vi "main.vi"() -> ()   [LabVIEW 2016]
uses:
  <vilib>/platform/TimedLoop/XDataNode/XDataNode.xnode
  <vilib>/Platform/TimedLoop/XDataNode/nitl_modes.ctl
  <vilib>/Platform/TimedLoop/XDataNode/XDNodeRunTimeDep.lvlib
  <vilib>/Platform/TimedLoop/XDataNode/wakeup.ctl
  <vilib>/Platform/TimedLoop/XDataNode/timing_clust.ctl
  <instrlib>/Lake Shore 425/Lake Shore 425.lvlib
panel:
  out "Temperature":dbl[](array[numeric])
  out "Multimeter":dbl[](array[numeric])
  out "Gaussmeter 3":dbl[](array[numeric])
  out "Gaussmeter 2":dbl[](array[numeric])
  out "Gaussmeter 1":dbl[](array[numeric])
  out "Status Multimeter":bool caption="Status"
  in  "Notes (must be entered before starting)":string
  in  "Multimeter\nMeasurement":u16(ring) caption="Measurement" items=["DC Voltage (50 A - 50 mV Shunt)", "DC Current (3 A Terminal)", "DC Current (10 A Terminal)", "AC Voltage (50 A - 50 mV Shunt)", "AC Current (3 A Terminal)", "AC Current (10 A Terminal)", "DC Voltage (other)", "AC Voltage (other)", "Continuity", "Diode", "Frequency", "Resistance 4-wire", "Period", "Resistance 2-wire", "Temperature", "DC Voltage Ratio", "Capacitance"]
  in  "VISA resource name Multimeter":refnum<visa-resource-name>
  in  "Switch Multimeter":bool
  out "Waveform Chart Multimeter":dbl(graph)
  in  "Temp. Monitor\nReadings per\nMeasurement":dbl caption="Temp. Monitor"
  in  "Multimeter\nReadings per\nMeasurement":dbl caption="Multimeter"
  in  "Readings per\nMeasurement":i32=5 caption="All Meters" min=1 step=1
  in  "Measure":bool
  out "z [mm]":dbl
  out "y [mm]":dbl
  out "x [mm]":dbl
  in  "Position File":path
  in  "Map Mode":bool
  in  "z":dbl caption="z [mm]"
  in  "y":dbl caption="y [mm]"
  in  "x":dbl caption="x [mm]"
  in  "Period [s]":dbl=1.0
  in  "Duration":dbl format="%<%H:%M:%S>t"
  out "XY Graph":cluster{dbl[], dbl[]}(graph)
  in  "Y-Axis":i32(ring)=6 items=["Time"=0, "x position"=1, "y position"=2, "z position"=3, "Gaussmeter 1"=4, "Gaussmeter 2"=6, "Gaussmeter 3"=8, "Multimeter"=10, "Temperature 1"=11, "Temperature 2"=12, "Temperature 3"=13, "Temperature 4"=14, "Temperature 5"=15, "Temperature 6"=16, "Temperature 7"=17, "Temperature 8"=18]
  in  "X-Axis":i32(ring)=4 items=["Time"=0, "x position"=1, "y position"=2, "z position"=3, "Gaussmeter 1"=4, "Gaussmeter 2"=6, "Gaussmeter 3"=8, "Multimeter"=10, "Temperature 1"=11, "Temperature 2"=12, "Temperature 3"=13, "Temperature 4"=14, "Temperature 5"=15, "Temperature 6"=16, "Temperature 7"=17, "Temperature 8"=18]
  in  "Moving Gaussmeter 3":bool caption="Moving"
  in  "x Gaussmeter 3":dbl caption="x [mm]"
  in  "y Gaussmeter 3":dbl caption="y [mm]"
  in  "z Gaussmeter 3":dbl caption="z [mm]"
  in  "Switch Gaussmeter 3":bool
  in  "VISA resource name Gaussmeter 3":refnum<visa-resource-name>
  out "Probe Type 3":u16(ring)=40 caption="Probe Type" items=["High Sensitivity"=40, "High Stability"=41, "Ultra-High Sensitivity"=42, "User Programmable Cable / High Sensitivity Probe"=50, "User Programmable Cable / High Stability Probe"=51, "User Programmable Cable / Ultra-High Sensitivity Probe"=52]
  out "Probe Serial Number 3":string caption="Probe Serial Number"
  out "Probe Sensitivity 3":dbl=0.001 caption="Probe Sensitivity" format="%^.3e"
  out "Field\nComp 3":bool caption="Field\nComp"
  out "Field Range  3":u16(ring)=1 caption="Field Range" items=["1 - Lowest"=1, "2"=2, "3"=3, "4 - Highest"=4]
  out "Field Units 3":u16(ring)=1 caption="Field Units" items=["Gauss"=1, "Tesla"=2, "Oersted"=3, "Amp/Meter"=4]
  out "Auto\nRange 3":bool caption="Auto\nRange"
  out "Status Gaussmeter 3":bool caption="Status"
  out "Waveform Chart Gaussmeter 3":dbl(graph)
  in  "Moving Gaussmeter 2":bool caption="Moving"
  in  "x Gaussmeter 2":dbl caption="x [mm]"
  in  "y Gaussmeter 2":dbl caption="y [mm]"
  in  "z Gaussmeter 2":dbl caption="z [mm]"
  in  "Switch Gaussmeter 2":bool
  in  "VISA resource name Gaussmeter 2":refnum<visa-resource-name>
  out "Probe Type 2":u16(ring)=40 caption="Probe Type" items=["High Sensitivity"=40, "High Stability"=41, "Ultra-High Sensitivity"=42, "User Programmable Cable / High Sensitivity Probe"=50, "User Programmable Cable / High Stability Probe"=51, "User Programmable Cable / Ultra-High Sensitivity Probe"=52]
  out "Probe Serial Number 2":string caption="Probe Serial Number"
  out "Probe Sensitivity 2":dbl=0.001 caption="Probe Sensitivity" format="%^.3e"
  out "Field\nComp 2":bool caption="Field\nComp"
  out "Field Range  2":u16(ring)=1 caption="Field Range" items=["1 - Lowest"=1, "2"=2, "3"=3, "4 - Highest"=4]
  out "Field Units 2":u16(ring)=1 caption="Field Units" items=["Gauss"=1, "Tesla"=2, "Oersted"=3, "Amp/Meter"=4]
  out "Auto\nRange 2":bool caption="Auto\nRange"
  out "Status Gaussmeter 2":bool caption="Status"
  out "Waveform Chart Gaussmeter 2":dbl(graph)
  in  "z Gaussmeter 1":dbl caption="z [mm]"
  in  "y Gaussmeter 1":dbl caption="y [mm]"
  in  "x Gaussmeter 1":dbl caption="x [mm]"
  in  "Moving Gaussmeter 1":bool caption="Moving"
  out "Status Gaussmeter 1":bool caption="Status"
  out "Auto\nRange":bool
  out "Field Units":u16(ring)=1 items=["Gauss"=1, "Tesla"=2, "Oersted"=3, "Amp/Meter"=4]
  out "Field Range":u16(ring)=1 items=["1 - Lowest"=1, "2"=2, "3"=3, "4 - Highest"=4]
  out "Field\nComp":bool
  out "Probe Sensitivity":dbl=0.001 format="%^.3e"
  out "Probe Serial Number":string
  out "Probe Type":u16(ring)=40 items=["High Sensitivity"=40, "High Stability"=41, "Ultra-High Sensitivity"=42, "User Programmable Cable / High Sensitivity Probe"=50, "User Programmable Cable / High Stability Probe"=51, "User Programmable Cable / Ultra-High Sensitivity Probe"=52]
  in  "VISA resource name Gaussmeter 1":refnum<visa-resource-name>
  in  "Switch Gaussmeter 1":bool
  out "Waveform Chart Gaussmeter 1":dbl(graph)
  out "Time [s]":dbl
  in  "Stop Button":bool
  out "Output File Name":string
  out "Output File Path":path
  in  "Output Folder Path":path=path "C:/Users/ephenix/Dropbox/Stony Brook Research Team Folder/LabVIEW/DATA_MegaVIEW"
  in  "VISA resource name Temperature Monitor":refnum<visa-resource-name>
  in  "Switch Temperature Monitor":bool
  out "Waveform Chart Temperature Monitor":dbl(graph)
  # "Multimeter (Agilent 34461A)"
  # "Readings per"
  # "Measurement"
  # "Timed MeasurementSettings"
  # "XY Graph Axes"
  # "Gaussmeter 3 (Lake Shore 425)"
  # "Gaussmeter 2 (Lake Shore 425)"
  # "Gaussmeter 1 (Lake Shore 425)"
  # "Temperature Monitor (Lake Shore 218)"
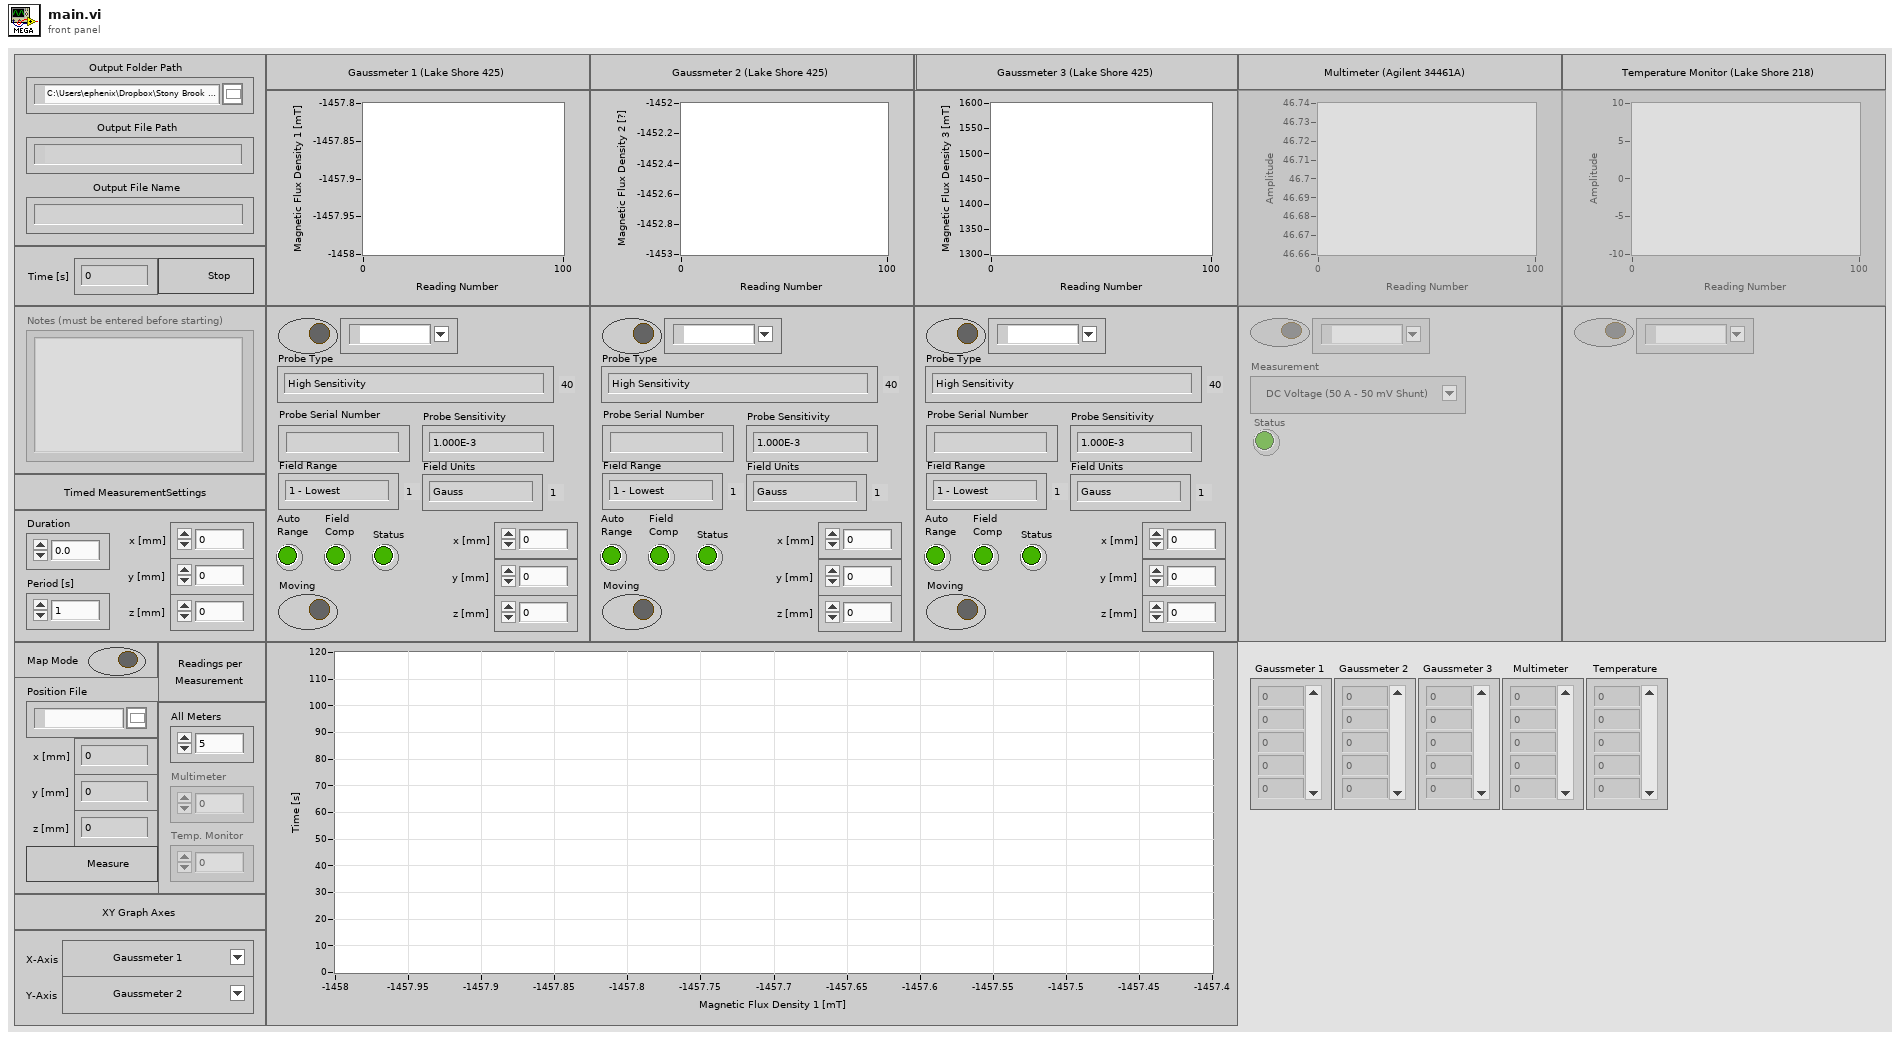
[diagram p1: front panel]
types:
  T1 = enum8{"Enabled", "Disabled", "Disabled and Grayed Out"}
  T2 = cluster{"VISA recourse name":refnum<visa-resource-name>, "switch":bool, "text":string, "units":i32, "status":bool}
  T3 = cluster{"VISA recourse name":cluster{refnum<visa-resource-name>, refnum<visa-resource-name>, refnum<visa-resource-name>, refnum<visa-resource-name>, refnum<visa-resource-name>}, "switch":cluster{bool, bool, bool, bool, bool}, "text":cluster{string, string, string, string, string}, "units":cluster{i32, i32, i32, i32, i32}}
  T4 = cluster{"VISA recourse name":refnum<visa-resource-name>, "VISA recourse name":refnum<visa-resource-name>, "VISA recourse name":refnum<visa-resource-name>, "VISA recourse name":refnum<visa-resource-name>, "VISA recourse name":refnum<visa-resource-name>}
  T5 = cluster{"switch":bool, "switch":bool, "switch":bool, "switch":bool, "switch":bool}
  T6 = cluster{"text":string, "text":string, "text":string, "text":string, "text":string}
  T7 = cluster{"units":i32, "units":i32, "units":i32, "units":i32, "units":i32}
  T8 = enum16{"open", "replace", "create", "open or create", "replace or create", "replace or create with confirmation"}
  T9 = typedef "XDNodeRunTimeDep.lvlib/timing_clust.ctl" = cluster{"Expected End [f-1]":u64, "Actual End [f-1]":u64, "Finished Late? [f-1]":bool, "Expected End [i-1]":u64, "Actual End [i-1]":u64, "Finished Late? [i-1]":bool, "Expected Start [i]":u64, "Actual Start [i]":u64, "Expected Start [f]":u64, "Actual Start [f]":u64, "Source Name":string, "Structure Name":string, "Period":i64, "Deadline":i64, "Offset":i64, "Start":i64, "Priority":i32, "Timeout":i32, "Mode":T10, "Wakeup Reason":T11, "Error":errorcluster, "Source Type":string, "Secondary Source Type":string, "Global End Time":u64, "Global Start Time":u64, "Frame Duration":u64, "Iteration Duration":u64, "Assigned CPU":i32, "I/O Scan Engine Mode":u32}
  T10 = typedef "XDNodeRunTimeDep.lvlib/nitl_modes.ctl" = enum32{"No Change", "Process missed periods, maintain original phase", "Discard missed periods, maintain original phase", "Process missed periods, ignore original phase", "Discard missed periods, ignore original phase"}
  T11 = typedef "XDNodeRunTimeDep.lvlib/wakeup.ctl" = enum32{"Normal", "Aborted", "Asynchronous wakeup", "Timing source error", "Timed loop error", "Timeout"}
  T12 = cluster{refnum<visa-resource-name>, refnum<visa-resource-name>, refnum<visa-resource-name>, refnum<visa-resource-name>, refnum<visa-resource-name>}
  T13 = cluster{"Field Reading":dbl, "Field Reading":dbl, "Field Reading":dbl, "Reading":dbl}
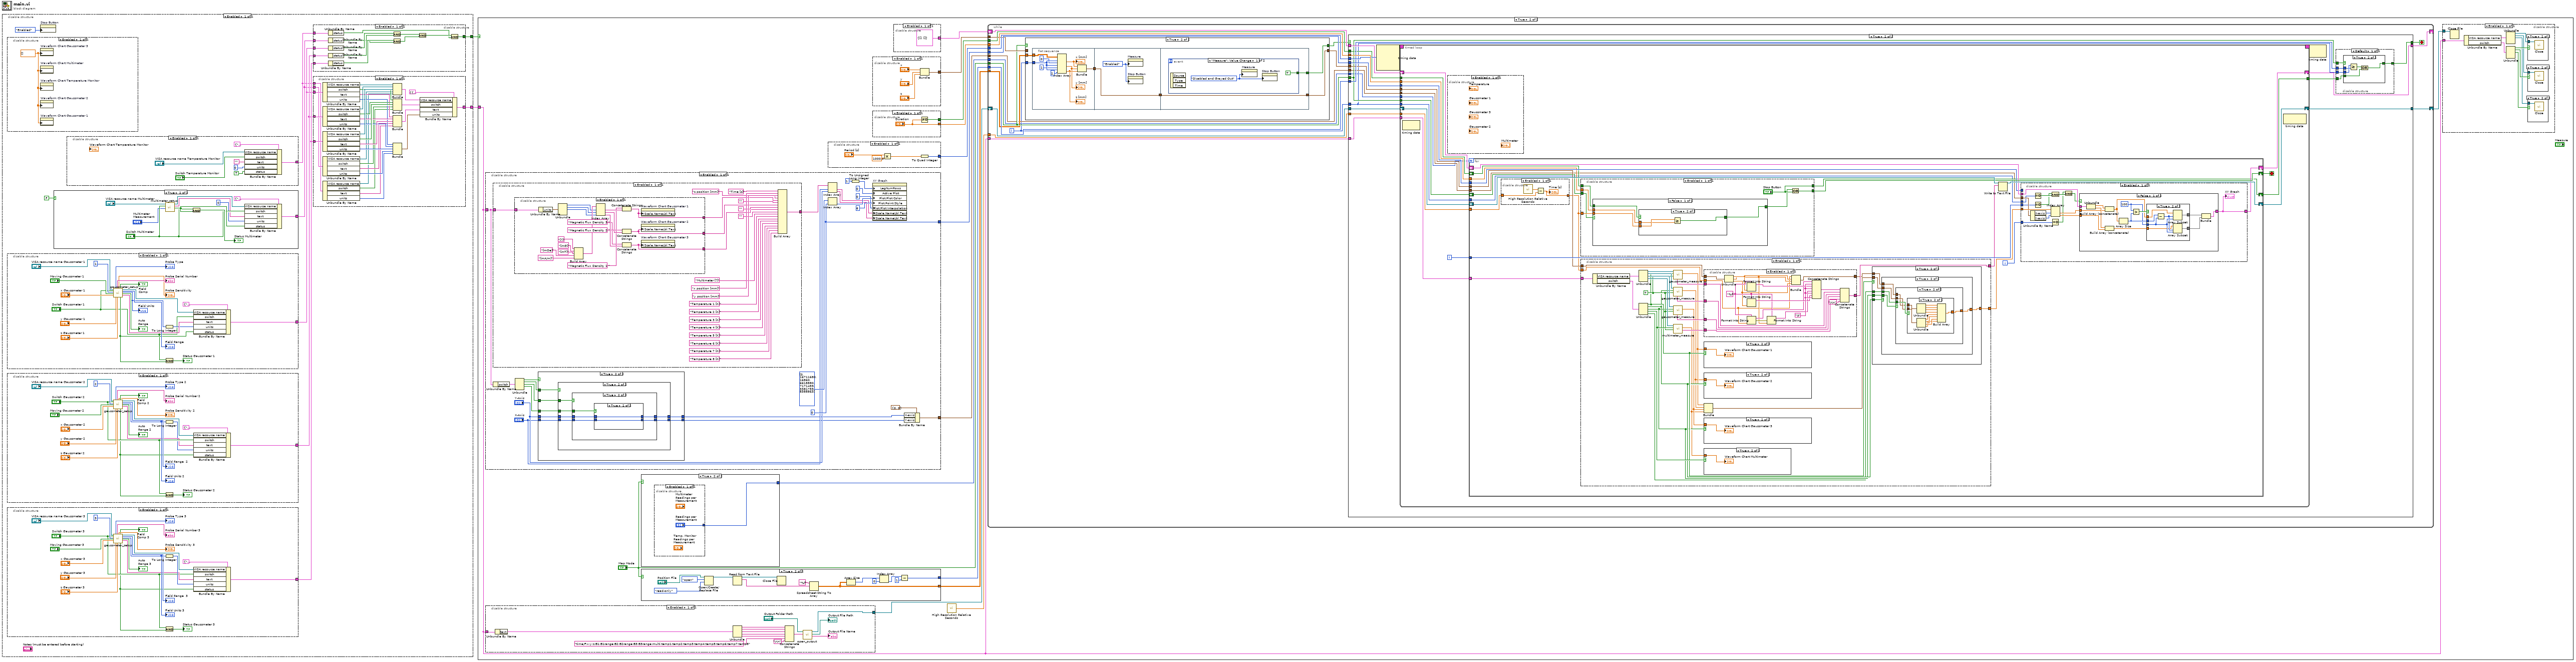
[diagram p0: block diagram]
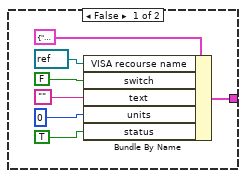
[diagram p2: hidden frame]
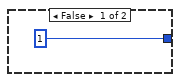
[diagram p4: hidden frame]
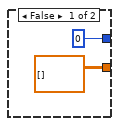
[diagram p12: hidden frame]
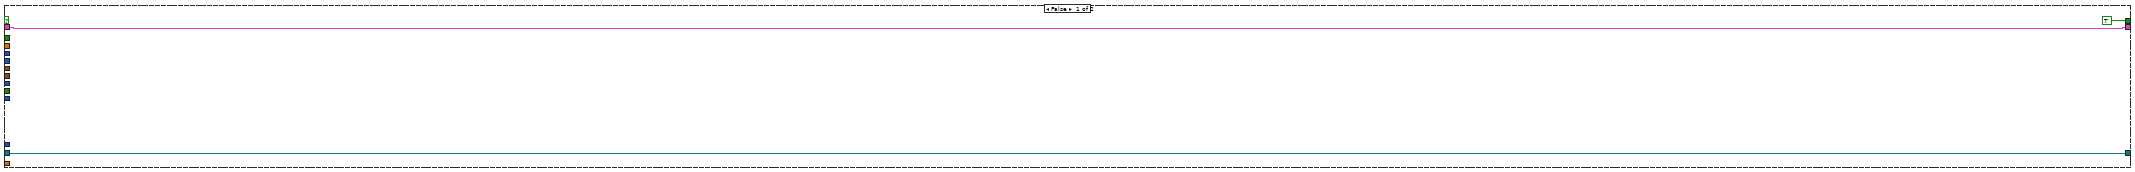
[diagram p13: hidden frame]
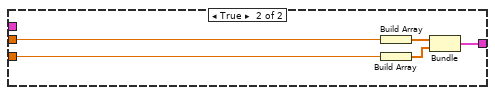
[diagram p15: hidden frame]
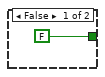
[diagram p16: hidden frame]
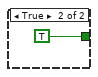
[diagram p17: hidden frame]
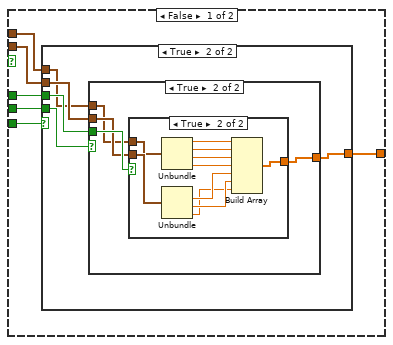
[diagram p18: hidden frame]
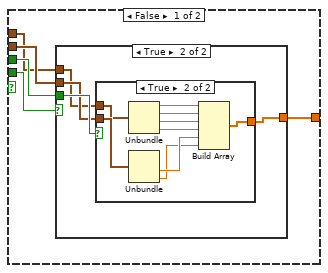
[diagram p19: hidden frame]
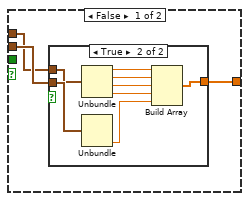
[diagram p20: hidden frame]
diagram:
  n1 = disable-structure shown="Enabled" {
    disable-tunnel: [w11] -> w2
    disable-tunnel: [w10] -> w1
    frame Enabled {
      n2 = disable-structure shown="Enabled" {
        frame Enabled {
          w36 = dbl[] [] ("History Data")
          n3 = property on="Waveform Chart Gaussmeter 3" class="WFChart (strict)"("History Data"=w36) -> ()  [unwired: 2 in, 2 out]
          n4 = property on="Waveform Chart Multimeter" class="WFChart (strict)"("History Data"=w36) -> ()  [unwired: 2 in, 2 out]
          n5 = property on="Waveform Chart Temperature Monitor" class="WFChart (strict)"("History Data"=w36) -> ()  [unwired: 2 in, 2 out]
          n6 = property on="Waveform Chart Gaussmeter 2" class="WFChart (strict)"("History Data"=w36) -> ()  [unwired: 2 in, 2 out]
          n7 = property on="Waveform Chart Gaussmeter 1" class="WFChart (strict)"("History Data"=w36) -> ()  [unwired: 2 in, 2 out]
        }
      }
      n8 = disable-structure shown="Enabled" {
        disable-tunnel: [w82] -> w8
        frame Enabled {
          n9 = call "gaussmeter_setup.vi"("VISA resource name Gaussmeter"="VISA resource name Gaussmeter 1", "Switch Gaussmeter"="Switch Gaussmeter 1", "Gaussmeter Number"=u8 1, "Moving Gaussmeter"="Moving Gaussmeter 1", "x Gaussmeter"="x Gaussmeter 1", "y Gaussmeter"="y Gaussmeter 1", "z Gaussmeter"="z Gaussmeter 1") -> ("Probe Type"=→"Probe Type":u16, "Probe Serial Number"=→"Probe Serial Number":string, "Probe Sensitivity"=→"Probe Sensitivity":dbl, "Probe Field\nCompensation On"=→"Field\nComp":bool, "Status Gaussmeter"=w80:bool, "Gaussmeter VISA resource name out"=w85:refnum<visa-resource-name>, "Field Range"=→"Field Range":u16, "Field Units"=w86:u16, "Auto Range On"=→"Auto\nRange":bool, "Text Output"=w84:string)  [unwired: 2 in, 1 out]
          "Field Units" <- w86
          n10 = To Long Integer(number=w86) -> (32bit integer=w83:i32)
          n11 = And(x="Switch Gaussmeter 1", y=w80) -> (x .and. y?=→"Status Gaussmeter 1":bool)
          n12 = Bundle By Name(cluster=T2 {"VISA recourse name"="", "switch"=TRUE, "text"="", "units"=0, "status"=TRUE} ("input cluster"), "VISA recourse name"=w85, "switch"="Switch Gaussmeter 1", "text"=w84, "units"=w83, "status"=w80) -> (w82:T2)
        }
      }
      n13 = disable-structure shown="Enabled" {
        disable-tunnel: [w58] -> w7
        frame Enabled {
          n14 = call "gaussmeter_setup.vi"("VISA resource name Gaussmeter"="VISA resource name Gaussmeter 2", "Switch Gaussmeter"="Switch Gaussmeter 2", "Gaussmeter Number"=u8 2, "Moving Gaussmeter"="Moving Gaussmeter 2", "x Gaussmeter"="x Gaussmeter 2", "y Gaussmeter"="y Gaussmeter 2", "z Gaussmeter"="z Gaussmeter 2") -> ("Probe Type"=→"Probe Type 2":u16, "Probe Serial Number"=→"Probe Serial Number 2":string, "Probe Sensitivity"=→"Probe Sensitivity 2":dbl, "Probe Field\nCompensation On"=→"Field\nComp 2":bool, "Status Gaussmeter"=w59:bool, "Gaussmeter VISA resource name out"=w63:refnum<visa-resource-name>, "Field Range"=→"Field Range  2":u16, "Field Units"=w65:u16, "Auto Range On"=→"Auto\nRange 2":bool, "Text Output"=w61:string)  [unwired: 2 in, 1 out]
          "Field Units 2" <- w65
          n15 = To Long Integer(number=w65) -> (32bit integer=w60:i32)
          n16 = And(x="Switch Gaussmeter 2", y=w59) -> (x .and. y?=→"Status Gaussmeter 2":bool)
          n17 = Bundle By Name(cluster=T2 {"VISA recourse name"="", "switch"=TRUE, "text"="", "units"=0, "status"=TRUE} ("input cluster"), "VISA recourse name"=w63, "switch"="Switch Gaussmeter 2", "text"=w61, "units"=w60, "status"=w59) -> (w58:T2)
        }
      }
      n18 = disable-structure shown="Enabled" {
        disable-tunnel: [w37] -> w9
        frame Enabled {
          n19 = call "gaussmeter_setup.vi"("VISA resource name Gaussmeter"="VISA resource name Gaussmeter 3", "Switch Gaussmeter"="Switch Gaussmeter 3", "Gaussmeter Number"=u8 3, "Moving Gaussmeter"="Moving Gaussmeter 3", "x Gaussmeter"="x Gaussmeter 3", "y Gaussmeter"="y Gaussmeter 3", "z Gaussmeter"="z Gaussmeter 3") -> ("Probe Type"=→"Probe Type 3":u16, "Probe Serial Number"=→"Probe Serial Number 3":string, "Probe Sensitivity"=→"Probe Sensitivity 3":dbl, "Probe Field\nCompensation On"=→"Field\nComp 3":bool, "Status Gaussmeter"=w38:bool, "Gaussmeter VISA resource name out"=w41:refnum<visa-resource-name>, "Field Range"=→"Field Range  3":u16, "Field Units"=w44:u16, "Auto Range On"=→"Auto\nRange 3":bool, "Text Output"=w42:string)  [unwired: 2 in, 1 out]
          "Field Units 3" <- w44
          n20 = To Long Integer(number=w44) -> (32bit integer=w43:i32)
          n21 = And(x="Switch Gaussmeter 3", y=w38) -> (x .and. y?=→"Status Gaussmeter 3":bool)
          n22 = Bundle By Name(cluster=T2 {"VISA recourse name"="", "switch"=TRUE, "text"="", "units"=0, "status"=TRUE} ("input cluster"), "VISA recourse name"=w41, "switch"="Switch Gaussmeter 3", "text"=w42, "units"=w43, "status"=w38) -> (w37:T2)
        }
      }
      n23 = property on="Stop Button" class="Bool"("DisabledEnum"=T1."Enabled" ("Disabled")) -> ()  [unwired: 2 in, 2 out]
      n24 = case shown="True" FALSE {
        tunnel: [w17 w19] -> w5
        frame False {
          n25 = Bundle By Name(cluster=T2 {"VISA recourse name"="", "switch"=TRUE, "text"="", "units"=0, "status"=TRUE} ("input cluster"), "VISA recourse name"=refnum<visa-resource-name> refnum, "switch"=FALSE, "text"="", "units"=0, "status"=TRUE) -> (w17:T2)
        }
        frame True {
          n26 = call "multimeter_setup.vi"("Measurement"="Multimeter\nMeasurement", "Switch"="Switch Multimeter", "VISA resource name"="VISA resource name Multimeter") -> ("status"=w27:bool, "text"=w23:string, "VISA resource name out"=w22:refnum<visa-resource-name>)  [unwired: 5 in, 1 out]
          n27 = And(x="Switch Multimeter", y=w27) -> (x .and. y?=→"Status Multimeter":bool)
          n28 = Bundle By Name(cluster=T2 {"VISA recourse name"="", "switch"=TRUE, "text"="", "units"=0, "status"=TRUE} ("input cluster"), "VISA recourse name"=w22, "switch"="Switch Multimeter", "text"=w23, "units"=0, "status"=w27) -> (w19:T2)
        }
      }
      n29 = disable-structure shown="Enabled" {
        disable-tunnel: [w32] -> w6
        frame Enabled {
          n30 = Bundle By Name(cluster=T2 {"VISA recourse name"="", "switch"=TRUE, "text"="", "units"=0, "status"=TRUE} ("input cluster"), "VISA recourse name"="VISA resource name Temperature Monitor", "switch"="Switch Temperature Monitor", "text"="", "units"=0, "status"=TRUE) -> (w32:T2)
        }
      }
      n31 = disable-structure shown="Enabled" {
        disable-tunnel: [w131] -> w11
        disable-tunnel: w9 -> [w139]
        disable-tunnel: w8 -> [w143]
        disable-tunnel: w7 -> [w140]
        disable-tunnel: w6 -> [w137]
        disable-tunnel: w5 -> [w138]
        frame Enabled {
          n32 = Unbundle By Name(w137) -> ("status"=w132:bool)
          n33 = Unbundle By Name(w138) -> ("status"=w135:bool)
          n34 = Unbundle By Name(w143) -> ("status"=w141:bool)
          n35 = Unbundle By Name(w140) -> ("status"=w142:bool)
          n36 = Unbundle By Name(w139) -> ("status"=w136:bool)
          n37 = And(x=w141, y=w142) -> (x .and. y?=w144:bool)
          n38 = And(x=w136, y=w135) -> (x .and. y?=w134:bool)
          n39 = And(x=w144, y=w134) -> (x .and. y?=w133:bool)
          n40 = And(x=w133, y=w132) -> (x .and. y?=w131:bool)
        }
      }
      n41 = disable-structure shown="Enabled" {
        disable-tunnel: [w126] -> w10
        disable-tunnel: w8 -> [w125]
        disable-tunnel: w7 -> [w123]
        disable-tunnel: w9 -> [w124]
        disable-tunnel: w5 -> [w109]
        disable-tunnel: w6 -> [w108]
        frame Enabled {
          n42 = Unbundle By Name(w125) -> ("VISA recourse name"=w122:refnum<visa-resource-name>, "switch"=w118:bool, "text"=w116:string, "units"=w111:i32)
          n43 = Unbundle By Name(w123) -> ("VISA recourse name"=w121:refnum<visa-resource-name>, "switch"=w119:bool, "text"=w115:string, "units"=w112:i32)
          n44 = Unbundle By Name(w124) -> ("VISA recourse name"=w120:refnum<visa-resource-name>, "switch"=w117:bool, "text"=w114:string, "units"=w113:i32)
          n45 = Unbundle By Name(w109) -> ("VISA recourse name"=w100:refnum<visa-resource-name>, "switch"=w103:bool, "text"=w104:string, "units"=w107:i32)
          n46 = Unbundle By Name(w108) -> ("VISA recourse name"=w101:refnum<visa-resource-name>, "switch"=w102:bool, "text"=w105:string, "units"=w106:i32)
          n47 = Bundle("VISA recourse name"=w122, "VISA recourse name"=w121, "VISA recourse name"=w120, "VISA recourse name"=w100, "VISA recourse name"=w101) -> (w130:T4)  [unwired: 1 in]
          n48 = Bundle("switch"=w118, "switch"=w119, "switch"=w117, "switch"=w103, "switch"=w102) -> (w129:T5)  [unwired: 1 in]
          n49 = Bundle("text"=w116, "text"=w115, "text"=w114, "text"=w104, "text"=w105) -> (w128:T6)  [unwired: 1 in]
          n50 = Bundle("units"=w111, "units"=w112, "units"=w113, "units"=w107, "units"=w106) -> (w127:T7)  [unwired: 1 in]
          n51 = Bundle By Name(cluster=T3 {"VISA recourse name"={"", "", "", "", ""}, "switch"={TRUE, TRUE, TRUE, TRUE, TRUE}, "text"={"", "", "", "", ""}, "units"={0, 0, 0, 0, 0}}, "VISA recourse name"=w130, "switch"=w129, "text"=w128, "units"=w127) -> (w126:T3)
        }
      }
    }
  }
  n52 = case shown="True" w2 {
    tunnel: w1 -> [_ w150]
    frame False {
    }
    frame True {
      n53 = disable-structure shown="Enabled" {
        disable-tunnel: [w208] -> w155
        disable-tunnel: w150 -> [w195]
        disable-tunnel: [w196] -> w151
        frame Enabled {
          w208 = 0
          n54 = disable-structure shown="Enabled" {
            disable-tunnel: [w245] -> w198
            disable-tunnel: w195 -> [w229]
            frame Enabled {
              n55 = disable-structure shown="Enabled" {
                disable-tunnel: [w257] -> w232
                disable-tunnel: [w256] -> w231
                disable-tunnel: [w255] -> w230
                disable-tunnel: w229 -> [w254]
                frame Enabled {
                  n56 = Unbundle By Name(w254) -> ("units"=w253:cluster{i32, i32, i32, i32, i32})
                  n57 = Unbundle(w253) -> (w252:i32, w251:i32, w250:i32)  [unwired: 2 out]
                  n58 = Build Array("[?]", "[mG]", "[mT]", "[mOe]", "[mA/m]") -> (w264:string[])
                  n59 = Index Array(array=w264, index #1=w252, index #2=w251, index #3=w250) -> (element #1=w261:string, element #2=w262:string, element #3=w263:string)
                  n60 = Concatenate Strings("Magnetic Flux Density 1 ", w261) -> (w255:string)
                  n61 = Concatenate Strings("Magnetic Flux Density 2 ", w262) -> (w256:string)
                  n62 = Concatenate Strings("Magnetic Flux Density 3 ", w263) -> (w257:string)
                  n63 = property on="Waveform Chart Gaussmeter 1" class="WFChart (strict)"("YScale.NameLbl.Text"=w255) -> ()  [unwired: 2 in, 2 out]
                  n64 = property on="Waveform Chart Gaussmeter 2" class="WFChart (strict)"("YScale.NameLbl.Text"=w256) -> ()  [unwired: 2 in, 2 out]
                  n65 = property on="Waveform Chart Gaussmeter 3" class="WFChart (strict)"("YScale.NameLbl.Text"=w257) -> ()  [unwired: 2 in, 2 out]
                }
              }
              n66 = Build Array("Time [s]", "x position [mm]", "y position [mm]", "z position [mm]", w230, "", w231, "", w232, "", "Multimeter [?]", "Temperature 1 [K]", "Temperature 2 [K]", "Temperature 3 [K]", "Temperature 4 [K]", "Temperature 5 [K]", "Temperature 6 [K]", "Temperature 7 [K]", "Temperature 8 [K]") -> (w245:string[])
            }
          }
          n67 = Unbundle By Name(w195) -> ("switch"=w194:cluster{bool, bool, bool, bool, bool})
          n68 = Unbundle(w194) -> (w193:bool, w192:bool, w191:bool, w190:bool)  [unwired: 1 out]
          n69 = case shown="True" w193 {
            tunnel: w192 -> [_ w215]
            tunnel: w191 -> [_ w214]
            tunnel: w190 -> [_ w213]
            tunnel: "Y-Axis" -> [_ w212]
            tunnel: "X-Axis" -> [_ w211]
            tunnel: [_ w210] -> w187
            tunnel: [_ w209] -> w186
            frame False {
            }
            frame True {
              n70 = case shown="True" w215 {
                tunnel: w214 -> [_ w221]
                tunnel: w213 -> [_ w220]
                tunnel: w212 -> [_ w219]
                tunnel: w211 -> [_ w218]
                tunnel: [_ w217] -> w210
                tunnel: [_ w216] -> w209
                frame False {
                }
                frame True {
                  n71 = case shown="True" w221 {
                    tunnel: w220 -> [_ w226]
                    tunnel: w219 -> [_ w225]
                    tunnel: w218 -> [_ w224]
                    tunnel: [_ w223] -> w217
                    tunnel: [_ w222] -> w216
                    frame False {
                    }
                    frame True {
                      n72 = case shown="True" w226 {
                        tunnel: w225 -> [_ w228]
                        tunnel: w224 -> [_ w227]
                        tunnel: [_ w228] -> w223
                        tunnel: [_ w227] -> w222
                        frame False {
                        }
                        frame True {
                        }
                      }
                    }
                  }
                }
              }
            }
          }
          n73 = Index Array(array=w198, index #1="X-Axis", index #2="Y-Axis") -> (element #1=w200:string, element #2=w199:string)
          n74 = Index Array(array=u32[] [0, 16711680, 16860, 6618880, 7171459, 3381759, 8388863], index=w208) -> (element=w206:u32)
          n75 = To Unsigned Long Integer(number=1 ("dimension size")) -> (unsigned 32bit integer=w203:u32)
          n76 = property on="XY Graph" class="XYGraph (strict)"("LegNumRows"=w203, "Active Plot"=u32 0, "Plot.Plot Color"=w206, "Plot.Point Style"=u8 6, "Plot.Plot Interpolation"=u8 0, "XScale.NameLbl.Text"=w200, "YScale.NameLbl.Text"=w199) -> ()  [unwired: 2 in, 2 out]
          n77 = Bundle By Name(cluster=cluster{"X-axis":i32, "Y-axis":i32} {"X-axis"=0, "Y-axis"=0}, "X-axis"=w187, "Y-axis"=w186) -> (w196:cluster{"X-axis":i32, "Y-axis":i32})
        }
      }
      n78 = disable-structure shown="Enabled" {
        disable-tunnel: [w281] -> w159
        disable-tunnel: w150 -> [w274]
        frame Enabled {
          n79 = Unbundle By Name(w274) -> ("text"=w275:cluster{string, string, string, string, string})
          n80 = Unbundle(w275) -> (w280:string, w279:string, w278:string, w272:string, w271:string)
          n81 = Concatenate Strings(w280, w279, w278, w272, w271, "time/F:x:y:z:B1:B1range:B2:B2range:B3:B3range:multi:temp1:temp2:temp3:temp4:temp5:temp6:temp7:temp8", "\r\n") -> (w282:string)
          n82 = call "open_output.vi"("Output File Header"=w282, "Output Folder Path"="Output Folder Path") -> ("Output File Name"=→"Output File Name":string, "Output File Path"=→"Output File Path":path, "refnum out"=w281:refnum<file>)  [unwired: 7 in]
        }
      }
      n83 = case shown="True" "Map Mode" {
        tunnel: [1 ("Gaussmeter\nReadings per\nMeasurement") w161] -> w146
        frame False {
        }
        frame True {
          n84 = disable-structure shown="Enabled" {
            disable-tunnel: ["Readings per\nMeasurement"] -> w161
            frame Enabled {
            }
          }
        }
      }
      n85 = case shown="True" "Map Mode" {
        tunnel: [0 w288] -> w154
        tunnel: [dbl[][] [] w287] -> w153
        frame False {
        }
        frame True {
          n86 = Open/Create/Replace File(file path (use dialog)="Position File", operation (0:open)=T8."open", access (0:read/write)=enum16{"read/write", "read-only", "write-only"}."read-only") -> (refnum out=w297:refnum<file>)  [unwired: 3 in, 2 out]
          n87 = Read from Text File(file (use dialog)=w297) -> (refnum out=w296:refnum<file>, text=w295:string)  [unwired: 3 in, 2 out]
          n88 = Close File(refnum=w296) -> ()  [unwired: 1 in, 2 out]
          n89 = Spreadsheet String To Array(format string="%f", spreadsheet string=w295) -> (array=w287:dbl[][])  [unwired: 2 in]
          n90 = Array Size(array=w287) -> (size(s)=w292:i32[])
          n91 = Index Array(array=w292, index=0) -> (element=w290:i32)
          n92 = Subtract(x=w290, y=1) -> (x-y=w288:i32)
        }
      }
      n93 = disable-structure shown="Enabled" {
        disable-tunnel: [w185] -> w157
        frame Enabled {
          n94 = Multiply(x="Period [s]", y=1000.0) -> (x*y=w182:dbl)
          n95 = To Quad Integer(1:w182) -> (0:w185:i64)
        }
      }
      n96 = disable-structure shown="Enabled" {
        disable-tunnel: [w178] -> w152
        frame Enabled {
          n97 = Bundle("x"="x", "y"="y", "z"="z") -> (w178:cluster{"x":dbl, "y":dbl, "z":dbl})  [unwired: 1 in]
        }
      }
      n98 = disable-structure shown="Enabled" {
        disable-tunnel: [w164] -> w148
        disable-tunnel: ["Duration"] -> w147
        frame Enabled {
          n99 = Not Equal To 0?(x="Duration") -> (x != 0?=w164:bool)
        }
      }
      n100 = disable-structure shown="Enabled" {
        disable-tunnel: [cluster{dbl[], dbl[]} {[], []}] -> w156
        frame Enabled {
        }
      }
      n101 = call <vilib>:"High Resolution Relative Seconds.vi"() -> ("relative seconds"=w158:dbl)
      n102 = while {
        tunnel: w158 -> [w317]
        tunnel: w148 -> [w306]
        tunnel: w147 -> [w316]
        tunnel: w157 -> [w315]
        tunnel: w155 -> [w313]
        tunnel: "Map Mode" -> [w308]
        shift-right: [w318] -> w149
        shift-left: w159 -> [w319]
        tunnel: w154 -> [w311]
        tunnel: w153 -> [w307]
        tunnel: w152 -> [w309]
        shift-right: [w305] -> _
        shift-left: w156 -> [w314]
        tunnel: w151 -> [w303]
        tunnel: w150 -> [w304]
        tunnel: w146 -> [w300]
        i -> [w302]
        stop <- w312 stop-if-true
        n103 = case shown="True" w308 {
          tunnel: w307 -> [_ w720]
          tunnel: [w714 w719] -> w310
          tunnel: w309 -> [w714 _]
          tunnel: w302 -> [_ w718]
          tunnel: [TRUE w715] -> w301
          frame False {
          }
          frame True {
            n104 = flat-sequence {
              tunnel: w720 -> [w729]
              tunnel: w718 -> [w724]
              tunnel: [w728] -> w717
              tunnel: w717 -> [w731]
              tunnel: [w731] -> w716
              tunnel: [w733] -> w719
              tunnel: w716 -> [w733]
              tunnel: [w732] -> w715
              frame #0 {
                n105 = Index Array(array=w729, index (row) #1=w724, index (col) #1=0 ("disabled index (col)"), index (row) #2=w724, index (col) #2=1 ("disabled index (col)"), index (row) #3=w724, index (col) #3=2 ("disabled index (col)")) -> (element #1=w725:dbl, element #2=w726:dbl, element #3=w727:dbl)
                "x [mm]" <- w725
                "y [mm]" <- w726
                "z [mm]" <- w727
                n106 = Bundle(w725, w726, w727) -> (w728:cluster{dbl, dbl, dbl})  [unwired: 1 in]
              }
              frame #1 {
                w730 = T1."Enabled" ("Disabled")
                n107 = property on="Measure" class="Bool"("DisabledEnum"=w730) -> ()  [unwired: 2 in, 2 out]
                n108 = property on="Stop Button" class="Bool"("DisabledEnum"=w730) -> ()  [unwired: 2 in, 2 out]
              }
              frame #2 {
                n109 = event shown="[0] \"Measure\": Value Change" {
                  selector: _ -> [_ _]
                  dyn-events: _ -> [_ _]
                  timeout: _ -> [_ _]
                  tunnel: [TRUE FALSE] -> w732
                  event "Measure": Value Change {
                    w734 = T1."Disabled and Grayed Out" ("Disabled")
                    n110 = event-data() -> ()  [unwired: 1 in, 3 out]
                    n111 = property on="Measure" class="Bool"("DisabledEnum"=w734) -> ()  [unwired: 2 in, 2 out]
                    n112 = property on="Stop Button" class="Bool"("DisabledEnum"=w734) -> ()  [unwired: 2 in, 2 out]
                  }
                  event "Stop Button": Value Change {
                    n113 = event-data() -> ()  [unwired: 1 in, 3 out]
                  }
                }
              }
            }
          }
        }
        n114 = case shown="True" w301 {
          tunnel: w319 -> [w321 w340]
          tunnel: [w321 w339] -> w318
          tunnel: w317 -> [_ w338]
          tunnel: w316 -> [_ w337]
          tunnel: w315 -> [_ w336]
          tunnel: w314 -> [w322 w335]
          tunnel: w313 -> [_ w334]
          tunnel: [TRUE w332] -> w312
          tunnel: w311 -> [_ w331]
          tunnel: w310 -> [_ w330]
          tunnel: w308 -> [_ w329]
          tunnel: w306 -> [_ w328]
          tunnel: [w322 w327] -> w305
          tunnel: w304 -> [_ w326]
          tunnel: w303 -> [_ w325]
          tunnel: w302 -> [_ w324]
          tunnel: w300 -> [_ w323]
          frame False {
          }
          frame True {
            n115 = node-c288(w336) -> (w342:T9)  [unwired: 3 in]
            n116 = timed-loop {
              timing: w342 -> [_]
              timing-out: [_] -> w341
              shift-right: [w358] -> w339
              shift-left: w340 -> [w359]
              tunnel: w338 -> [w357]
              tunnel: w337 -> [w349]
              shift-right: [w352] -> w327
              shift-left: w335 -> [w354]
              tunnel: w334 -> [w353]
              tunnel: w329 -> [w348]
              tunnel: [w351] -> w333
              tunnel: w330 -> [w350]
              tunnel: w328 -> [w347]
              tunnel: w326 -> [w346]
              tunnel: w325 -> [w345]
              tunnel: w324 -> [w344]
              tunnel: w323 -> [w343]
              i -> [w355]
              stop <- w356 stop-if-true
              n117 = node-c288() -> ()  [unwired: 1 in, 1 out]
              n118 = disable-structure shown="Enabled" {
                frame Enabled {
                }
              }
              n119 = for {
                N: w343 -> [_]
                tunnel: w357 -> [w377]
                tunnel: w355 -> [w374]
                tunnel: w353 -> [w372]
                tunnel: w350 -> [w369]
                tunnel: w349 -> [w368]
                tunnel: w346 -> [w364]
                tunnel: w345 -> [w363]
                tunnel: w344 -> [w362]
                shift-right: [w378] -> w358
                shift-left: w359 -> [w379]
                shift-right: [w371] -> w352
                shift-left: w354 -> [w373]
                shift-right: [w370] -> w351
                shift-left: w348 -> [w366]
                shift-right: [w376] -> w356
                shift-left: w347 -> [w365]
                i -> [w361]
                n120 = disable-structure shown="Enabled" {
                  disable-tunnel: w377 -> [w440]
                  disable-tunnel: [w439] -> w367
                  frame Enabled {
                    n121 = call <vilib>:"High Resolution Relative Seconds.vi"() -> ("relative seconds"=w441:dbl)
                    n122 = Subtract(x=w441, y=w440) -> (x-y=w439:dbl)
                    "Time [s]" <- w439
                  }
                }
                n123 = disable-structure shown="Enabled" {
                  disable-tunnel: [w429] -> w376
                  disable-tunnel: ["Stop Button"] -> w370
                  disable-tunnel: w368 -> [w427]
                  disable-tunnel: w367 -> [w426]
                  disable-tunnel: w366 -> [w424]
                  disable-tunnel: w365 -> [w423]
                  frame Enabled {
                    n124 = case shown="False" w424 {
                      tunnel: w427 -> [w432 _]
                      tunnel: w426 -> [w431 _]
                      tunnel: w423 -> [w430 _]
                      tunnel: [w433 TRUE] -> w425
                      frame False {
                        n125 = case shown="True" w430 {
                          tunnel: w431 -> [_ w437]
                          tunnel: w432 -> [_ w436]
                          tunnel: [FALSE w435] -> w433
                          frame False {
                          }
                          frame True {
                            n126 = Greater Or Equal?(x=w437, y=w436) -> (x >= y?=w435:bool)
                          }
                        }
                      }
                      frame True {
                      }
                    }
                    n127 = Or(x=w425, y="Stop Button") -> (x .or. y?=w429:bool)
                  }
                }
                n128 = disable-structure shown="Enabled" {
                  disable-tunnel: [w452] -> w375
                  disable-tunnel: w369 -> [w468]
                  disable-tunnel: w367 -> [w453]
                  disable-tunnel: w364 -> [w467]
                  disable-tunnel: [w454] -> w360
                  frame Enabled {
                    w459 = TRUE ("Switch 1000x")
                    n129 = Unbundle By Name(w467) -> ("VISA recourse name"=w466:T12, "switch"=w465:cluster{bool, bool, bool, bool, bool})
                    n130 = Unbundle(w466) -> (w464:refnum<visa-resource-name>, w463:refnum<visa-resource-name>, w462:refnum<visa-resource-name>, w461:refnum<visa-resource-name>)  [unwired: 1 out]
                    n131 = Unbundle(w465) -> (w451:bool, w450:bool, w449:bool, w460:bool, w448:bool)
                    n132 = call "gaussmeter_measure.vi"("Switch 1000x"=w459, "Switch Gaussmeter"=w451, "VISA resource name"=w464) -> ("Field Reading"=w447:dbl, "output string"=w455:string)  [unwired: 3 in, 4 out]
                    n133 = call "gaussmeter_measure.vi"("Switch 1000x"=w459, "Switch Gaussmeter"=w450, "VISA resource name"=w463) -> ("Field Reading"=w446:dbl, "output string"=w456:string)  [unwired: 3 in, 4 out]
                    n134 = call "gaussmeter_measure.vi"("Switch 1000x"=w459, "Switch Gaussmeter"=w449, "VISA resource name"=w462) -> ("Field Reading"=w445:dbl, "output string"=w457:string)  [unwired: 3 in, 4 out]
                    n135 = call "multimeter_measure.vi"("Switch 1000x"=w459, "Switch Multimeter"=w460, "VISA resource name"=w461) -> ("String"=w458:string, "Reading"=w444:dbl)  [unwired: 5 in, 2 out]
                    n136 = disable-structure shown="Enabled" {
                      disable-tunnel: w468 -> [w692]
                      disable-tunnel: w458 -> [w687]
                      disable-tunnel: w457 -> [w691]
                      disable-tunnel: w456 -> [w690]
                      disable-tunnel: w455 -> [w689]
                      disable-tunnel: [w688] -> w454
                      disable-tunnel: w453 -> [w674]
                      disable-tunnel: [w673] -> w442
                      frame Enabled {
                        w678 = "%f" ("format string")
                        w685 = "\t"
                        n137 = Unbundle(w692) -> ("x"=w677:dbl, "y"=w676:dbl, "z"=w675:dbl)
                        n138 = Format Into String(format string=w678, w677) -> (resulting string=w680:string)  [unwired: 2 in, 1 out]
                        n139 = Format Into String(format string=w678, w675) -> (resulting string=w682:string)  [unwired: 2 in, 1 out]
                        n140 = Format Into String(format string=w678, w674) -> (resulting string=w679:string, error out=w683:errorcluster)  [unwired: 2 in]
                        n141 = Format Into String(format string=w678, error in=w683, w676) -> (resulting string=w681:string)  [unwired: 1 in, 1 out]
                        n142 = Bundle(w674, "x"=w677, "y"=w676, "z"=w675) -> (w673:cluster{dbl, "x":dbl, "y":dbl, "z":dbl})  [unwired: 1 in]
                        n143 = Concatenate Strings(w679, w685, w680, w685, w681, w685, w682, w685) -> (w684:string)
                        n144 = Concatenate Strings(w684, w689, w690, w691, w687, "\r\n") -> (w688:string)
                      }
                    }
                    n145 = case shown="True" w451 {
                      tunnel: w447 -> [_ w695]
                      frame False {
                      }
                      frame True {
                        "Waveform Chart Gaussmeter 1" <- w695
                      }
                    }
                    n146 = case shown="True" w450 {
                      tunnel: w446 -> [_ w694]
                      frame False {
                      }
                      frame True {
                        "Waveform Chart Gaussmeter 2" <- w694
                      }
                    }
                    n147 = Bundle("Field Reading"=w447, "Field Reading"=w446, "Field Reading"=w445, "Reading"=w444) -> (w443:T13)  [unwired: 1 in]
                    n148 = case shown="True" w449 {
                      tunnel: w445 -> [_ w693]
                      frame False {
                      }
                      frame True {
                        "Waveform Chart Gaussmeter 3" <- w693
                      }
                    }
                    n149 = case shown="True" w460 {
                      tunnel: w444 -> [_ w672]
                      frame False {
                      }
                      frame True {
                        "Waveform Chart Multimeter" <- w672
                      }
                    }
                    n150 = case shown="True" w451 {
                      tunnel: [w474 w571] -> w452
                      tunnel: w450 -> [w471 w570]
                      tunnel: w449 -> [w469 w569]
                      tunnel: w448 -> [w470 w568]
                      tunnel: w443 -> [w472 w567]
                      tunnel: w442 -> [w473 w566]
                      frame False {
                        n151 = case shown="True" w471 {
                          tunnel: [w475 w522] -> w474
                          tunnel: w469 -> [w478 w521]
                          tunnel: w470 -> [w479 w520]
                          tunnel: w472 -> [w477 w519]
                          tunnel: w473 -> [w476 w518]
                          frame False {
                            n152 = case shown="True" w478 {
                              tunnel: [w482 w500] -> w475
                              tunnel: w479 -> [_ w499]
                              tunnel: w477 -> [w481 w498]
                              tunnel: w476 -> [w480 w497]
                              frame False {
                                n153 = case shown="True" {
                                selector: _ -> [_ _]
                                tunnel: [w488 w495] -> w482
                                tunnel: w481 -> [_ w496]
                                tunnel: w480 -> [w487 w494]
                                frame False {
                                n154 = Unbundle(w487) -> (w483:dbl, "x"=w484:dbl, "y"=w485:dbl, "z"=w486:dbl)
                                n155 = Build Array(w483, w484, w485, w486) -> (w488:dbl[])
                                }
                                frame True {
                                n156 = Unbundle(w494) -> (w493:dbl, "x"=w492:dbl, "y"=w491:dbl, "z"=w490:dbl)
                                n157 = Unbundle(w496) -> ("Reading"=w489:dbl)  [unwired: 3 out]
                                n158 = Build Array(w493, w492, w491, w490, w489) -> (w495:dbl[])
                                }
                                }
                              }
                              frame True {
                                n159 = case shown="True" w499 {
                                tunnel: [w508 w516] -> w500
                                tunnel: w498 -> [w507 w517]
                                tunnel: w497 -> [w504 w515]
                                frame False {
                                n160 = Unbundle(w504) -> (w506:dbl, "x"=w505:dbl, "y"=w503:dbl, "z"=w502:dbl)
                                n161 = Unbundle(w507) -> ("Field Reading"=w501:dbl)  [unwired: 3 out]
                                n162 = Build Array(w506, w505, w503, w502, w501) -> (w508:dbl[])
                                }
                                frame True {
                                n163 = Unbundle(w515) -> (w514:dbl, "x"=w513:dbl, "y"=w512:dbl, "z"=w511:dbl)
                                n164 = Unbundle(w517) -> ("Field Reading"=w510:dbl, "Reading"=w509:dbl)  [unwired: 2 out]
                                n165 = Build Array(w514, w513, w512, w511, w510, w509) -> (w516:dbl[])
                                }
                                }
                              }
                            }
                          }
                          frame True {
                            n166 = case shown="True" w521 {
                              tunnel: [w525 w546] -> w522
                              tunnel: w520 -> [_ w545]
                              tunnel: w519 -> [w524 w544]
                              tunnel: w518 -> [w523 w543]
                              frame False {
                                n167 = case shown="True" {
                                selector: _ -> [_ _]
                                tunnel: [w533 w541] -> w525
                                tunnel: w524 -> [w532 w542]
                                tunnel: w523 -> [w531 w540]
                                frame False {
                                n168 = Unbundle(w531) -> (w530:dbl, "x"=w529:dbl, "y"=w528:dbl, "z"=w527:dbl)
                                n169 = Unbundle(w532) -> ("Field Reading"=w526:dbl)  [unwired: 3 out]
                                n170 = Build Array(w530, w529, w528, w527, w526) -> (w533:dbl[])
                                }
                                frame True {
                                n171 = Unbundle(w540) -> (w536:dbl, "x"=w537:dbl, "y"=w538:dbl, "z"=w539:dbl)
                                n172 = Unbundle(w542) -> ("Field Reading"=w535:dbl, "Reading"=w534:dbl)  [unwired: 2 out]
                                n173 = Build Array(w536, w537, w538, w539, w535, w534) -> (w541:dbl[])
                                }
                                }
                              }
                              frame True {
                                n174 = case shown="True" w545 {
                                tunnel: [w555 w564] -> w546
                                tunnel: w544 -> [w554 w565]
                                tunnel: w543 -> [w553 w563]
                                frame False {
                                n175 = Unbundle(w553) -> (w549:dbl, "x"=w550:dbl, "y"=w551:dbl, "z"=w552:dbl)
                                n176 = Unbundle(w554) -> ("Field Reading"=w547:dbl, "Field Reading"=w548:dbl)  [unwired: 2 out]
                                n177 = Build Array(w549, w550, w551, w552, w547, w548) -> (w555:dbl[])
                                }
                                frame True {
                                n178 = Unbundle(w563) -> (w562:dbl, "x"=w561:dbl, "y"=w560:dbl, "z"=w559:dbl)
                                n179 = Unbundle(w565) -> ("Field Reading"=w558:dbl, "Field Reading"=w557:dbl, "Reading"=w556:dbl)  [unwired: 1 out]
                                n180 = Build Array(w562, w561, w560, w559, w558, w557, w556) -> (w564:dbl[])
                                }
                                }
                              }
                            }
                          }
                        }
                      }
                      frame True {
                        n181 = case shown="True" w570 {
                          tunnel: [w572 w624] -> w571
                          tunnel: w569 -> [w575 w623]
                          tunnel: w568 -> [w576 w622]
                          tunnel: w567 -> [w574 w621]
                          tunnel: w566 -> [w573 w620]
                          frame False {
                            n182 = case shown="True" w575 {
                              tunnel: [w579 w600] -> w572
                              tunnel: w576 -> [_ w599]
                              tunnel: w574 -> [w578 w598]
                              tunnel: w573 -> [w577 w597]
                              frame False {
                                n183 = case shown="True" {
                                selector: _ -> [_ _]
                                tunnel: [w586 w595] -> w579
                                tunnel: w578 -> [w585 w596]
                                tunnel: w577 -> [w584 w593]
                                frame False {
                                n184 = Unbundle(w584) -> (w580:dbl, "x"=w581:dbl, "y"=w582:dbl, "z"=w583:dbl)
                                n185 = Unbundle(w585) -> ("Field Reading"=w587:dbl)  [unwired: 3 out]
                                n186 = Build Array(w580, w581, w582, w583, w587) -> (w586:dbl[])
                                }
                                frame True {
                                n187 = Unbundle(w593) -> (w592:dbl, "x"=w591:dbl, "y"=w590:dbl, "z"=w589:dbl)
                                n188 = Unbundle(w596) -> ("Field Reading"=w594:dbl, "Reading"=w588:dbl)  [unwired: 2 out]
                                n189 = Build Array(w592, w591, w590, w589, w594, w588) -> (w595:dbl[])
                                }
                                }
                              }
                              frame True {
                                n190 = case shown="True" w599 {
                                tunnel: [w608 w618] -> w600
                                tunnel: w598 -> [w607 w619]
                                tunnel: w597 -> [w603 w614]
                                frame False {
                                n191 = Unbundle(w603) -> (w605:dbl, "x"=w604:dbl, "y"=w602:dbl, "z"=w601:dbl)
                                n192 = Unbundle(w607) -> ("Field Reading"=w609:dbl, "Field Reading"=w606:dbl)  [unwired: 2 out]
                                n193 = Build Array(w605, w604, w602, w601, w609, w606) -> (w608:dbl[])
                                }
                                frame True {
                                n194 = Unbundle(w614) -> (w613:dbl, "x"=w612:dbl, "y"=w611:dbl, "z"=w610:dbl)
                                n195 = Unbundle(w619) -> ("Field Reading"=w617:dbl, "Field Reading"=w616:dbl, "Reading"=w615:dbl)  [unwired: 1 out]
                                n196 = Build Array(w613, w612, w611, w610, w617, w616, w615) -> (w618:dbl[])
                                }
                                }
                              }
                            }
                          }
                          frame True {
                            n197 = case shown="True" w623 {
                              tunnel: [w627 w650] -> w624
                              tunnel: w622 -> [_ w649]
                              tunnel: w621 -> [w626 w648]
                              tunnel: w620 -> [w625 w647]
                              frame False {
                                n198 = case shown="True" {
                                selector: _ -> [_ _]
                                tunnel: [w634 w645] -> w627
                                tunnel: w626 -> [w633 w646]
                                tunnel: w625 -> [w632 w641]
                                frame False {
                                n199 = Unbundle(w632) -> (w631:dbl, "x"=w630:dbl, "y"=w629:dbl, "z"=w628:dbl)
                                n200 = Unbundle(w633) -> ("Field Reading"=w635:dbl, "Field Reading"=w636:dbl)  [unwired: 2 out]
                                n201 = Build Array(w631, w630, w629, w628, w635, w636) -> (w634:dbl[])
                                }
                                frame True {
                                n202 = Unbundle(w641) -> (w637:dbl, "x"=w638:dbl, "y"=w639:dbl, "z"=w640:dbl)
                                n203 = Unbundle(w646) -> ("Field Reading"=w644:dbl, "Field Reading"=w643:dbl, "Reading"=w642:dbl)  [unwired: 1 out]
                                n204 = Build Array(w637, w638, w639, w640, w644, w643, w642) -> (w645:dbl[])
                                }
                                }
                              }
                              frame True {
                                n205 = case shown="True" w649 {
                                tunnel: [w657 w670] -> w650
                                tunnel: w648 -> [w656 w671]
                                tunnel: w647 -> [w655 w665]
                                frame False {
                                n206 = Unbundle(w655) -> (w651:dbl, "x"=w652:dbl, "y"=w653:dbl, "z"=w654:dbl)
                                n207 = Unbundle(w656) -> ("Field Reading"=w658:dbl, "Field Reading"=w659:dbl, "Field Reading"=w660:dbl)  [unwired: 1 out]
                                n208 = Build Array(w651, w652, w653, w654, w658, w659, w660) -> (w657:dbl[])
                                }
                                frame True {
                                n209 = Unbundle(w665) -> (w664:dbl, "x"=w663:dbl, "y"=w662:dbl, "z"=w661:dbl)
                                n210 = Unbundle(w671) -> ("Field Reading"=w669:dbl, "Field Reading"=w668:dbl, "Field Reading"=w667:dbl, "Reading"=w666:dbl)
                                n211 = Build Array(w664, w663, w662, w661, w669, w668, w667, w666) -> (w670:dbl[])
                                }
                                }
                              }
                            }
                          }
                        }
                      }
                    }
                  }
                }
                n212 = Write to Text File(file (use dialog)=w379, text=w360) -> (refnum out=w378:refnum<file>)  [unwired: 2 in, 2 out]
                n213 = disable-structure shown="Enabled" {
                  disable-tunnel: w375 -> [w395]
                  disable-tunnel: w374 -> [w388]
                  disable-tunnel: w373 -> [w392]
                  disable-tunnel: w372 -> [_]
                  disable-tunnel: [w380] -> w371
                  disable-tunnel: w363 -> [w389]
                  disable-tunnel: w362 -> [w385]
                  disable-tunnel: w361 -> [w381]
                  frame Enabled {
                    n214 = Unbundle By Name(w389) -> ("X-axis"=w391:i32, "Y-axis"=w390:i32)
                    n215 = Equal To 0?(x=w385) -> (x = 0?=w387:bool)
                    n216 = Equal To 0?(x=w388) -> (x = 0?=w386:bool)
                    n217 = And(x=w386, y=w387) -> (x .and. y?=w384:bool)
                    n218 = Equal To 0?(x=w381) -> (x = 0?=w382:bool)
                    n219 = Index Array(array=w395, index #1=w391, index #2=w390) -> (element #1=w394:dbl, element #2=w393:dbl)
                    n220 = And(x=w382, y=w384) -> (x .and. y?=w383:bool)
                    n221 = case shown="False" w383 {
                      tunnel: [w406 w420] -> w380
                      tunnel: w392 -> [w405 _]
                      tunnel: w393 -> [w403 w418]
                      tunnel: w394 -> [w404 w419]
                      frame False {
                        w400 = 100 ("x")
                        n222 = Unbundle(w405) -> (w407:dbl[], w408:dbl[])
                        n223 = Build Array (concatenate)(w407, w404) -> (w399:dbl[])
                        n224 = Build Array (concatenate)(w408, w403) -> (w397:dbl[])
                        n225 = Array Size(array=w399) -> (size(s)=w401:i32)
                        n226 = Greater?(x=w400, y=w401) -> (0:w402:bool)
                        n227 = case shown="True" w402 {
                          tunnel: w399 -> [w410 w417]
                          tunnel: w401 -> [_ w416]
                          tunnel: w400 -> [_ w414]
                          tunnel: [w410 w415] -> w398
                          tunnel: w397 -> [w409 w412]
                          tunnel: [w409 w411] -> w396
                          frame False {
                          }
                          frame True {
                            n228 = Subtract(x=w416, y=w414) -> (x-y=w413:i32)
                            n229 = Array Subset(array=w417, index=w413, length=w414) -> (w415:dbl[])
                            n230 = Array Subset(array=w412, index=w413, length=w414) -> (w411:dbl[])
                          }
                        }
                        n231 = Bundle(w398, w396) -> (w406:cluster{dbl[], dbl[]})  [unwired: 1 in]
                      }
                      frame True {
                        n232 = Build Array(w419) -> (w421:dbl[])
                        n233 = Build Array(w418) -> (w422:dbl[])
                        n234 = Bundle(w421, w422) -> (w420:cluster{dbl[], dbl[]})  [unwired: 1 in]
                      }
                    }
                    "XY Graph" <- w380
                  }
                }
              }
              n235 = node-c288() -> ()  [unwired: 1 in, 1 out]
            }
            n236 = node-c288(w341) -> ()  [unwired: 1 out]
            n237 = disable-structure shown="Default" {
              disable-tunnel: w333 -> [w706]
              disable-tunnel: [w705] -> w332
              disable-tunnel: w331 -> [w704]
              disable-tunnel: w324 -> [w703]
              disable-tunnel: w329 -> [w702]
              frame Enabled {
                n238 = case shown="True" w702 {
                  tunnel: w706 -> [_ w712]
                  tunnel: [TRUE w711] -> w705
                  tunnel: w704 -> [_ w710]
                  tunnel: w703 -> [_ w709]
                  frame False {
                  }
                  frame True {
                    n239 = Greater Or Equal?(x=w709, y=w710) -> (x >= y?=w708:bool)
                    n240 = Or(x=w708, y=w712) -> (x .or. y?=w711:bool)
                  }
                }
              }
            }
          }
        }
      }
      n241 = disable-structure shown="Enabled" {
        disable-tunnel: w150 -> [w170]
        disable-tunnel: w149 -> [w169]
        frame Enabled {
          n242 = Close File(refnum=w169) -> ()  [unwired: 1 in, 2 out]
          n243 = Unbundle By Name(w170) -> ("VISA recourse name"=w168:T12, "switch"=w174:cluster{bool, bool, bool, bool, bool})
          n244 = Unbundle(w168) -> (w165:refnum<visa-resource-name>, w166:refnum<visa-resource-name>, w167:refnum<visa-resource-name>)  [unwired: 2 out]
          n245 = Unbundle(w174) -> (w173:bool, w172:bool, w171:bool)  [unwired: 2 out]
          n246 = case shown="True" w173 {
            tunnel: w165 -> [_ w177]
            frame False {
            }
            frame True {
              n247 = call <instrlib>:"Close.vi"("VISA resource name"=w177) -> ()  [unwired: 10 in, 1 out]
            }
          }
          n248 = case shown="True" w172 {
            tunnel: w166 -> [_ w176]
            frame False {
            }
            frame True {
              n249 = call <instrlib>:"Close.vi"("VISA resource name"=w176) -> ()  [unwired: 10 in, 1 out]
            }
          }
          n250 = case shown="True" w171 {
            tunnel: w167 -> [_ w175]
            frame False {
            }
            frame True {
              n251 = call <instrlib>:"Close.vi"("VISA resource name"=w175) -> ()  [unwired: 10 in, 1 out]
            }
          }
        }
      }
    }
  }
